vi "testVI.vi"() -> ()   [LabVIEW 2018]
uses:
  pgfPlotAxis_t.ctl
  <vilib>/Waveform/WDTOps.llb/WDT Get Waveform Time Array DBL.vi
  <vilib>/measure/NI_MABase.lvlib
panel:
  out "output LaTeX":string
  in  "standard deviation":dbl=1.0 format="%.2p"
  out "Waveform Graph":waveform(dbl)[](graph)=[{"t0"=timestamp(0 s since 1904-01-01), "dt"=0.001, "Y"=array[1000 elements]}, {"t0"=timestamp(0 s since 1904-01-01), "dt"=0.001, "Y"=array[1000 elements]}]
  in  "Frequency":dbl(slide)=1.9083969465648856 scale=0.0..10.0
  in  "Amplitude":dbl(slide)=3.5114503816793894 scale=0.0..10.0
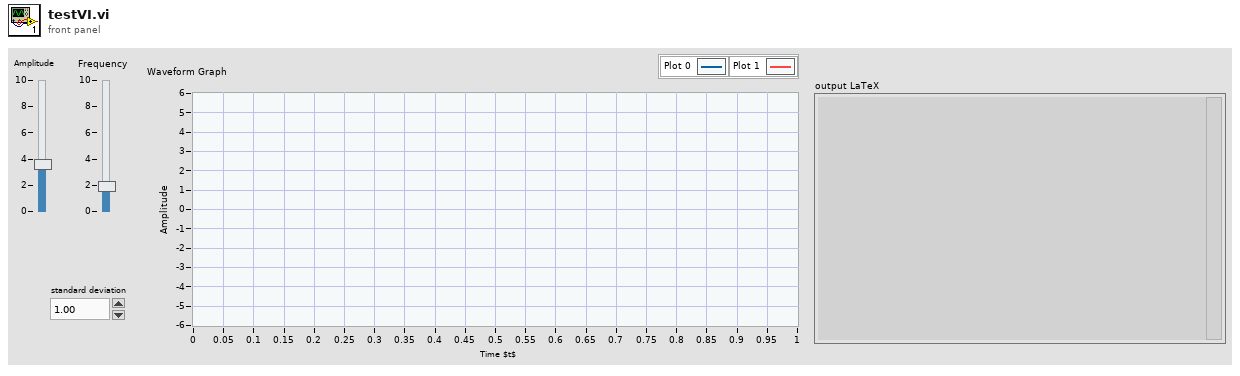
[diagram p1: front panel]
types:
  T1 = typedef "pgfPlotAxis_t.ctl" = cluster{"x values":dbl[], "y values":dbl[], "xmin":dbl, "xmax":dbl, "ymin":dbl, "ymax":dbl, "Line Style":u8, "Line Width":u8, "Plot Color":u32, "Point Style":u8, "xLabel":string, "yLabel":string}
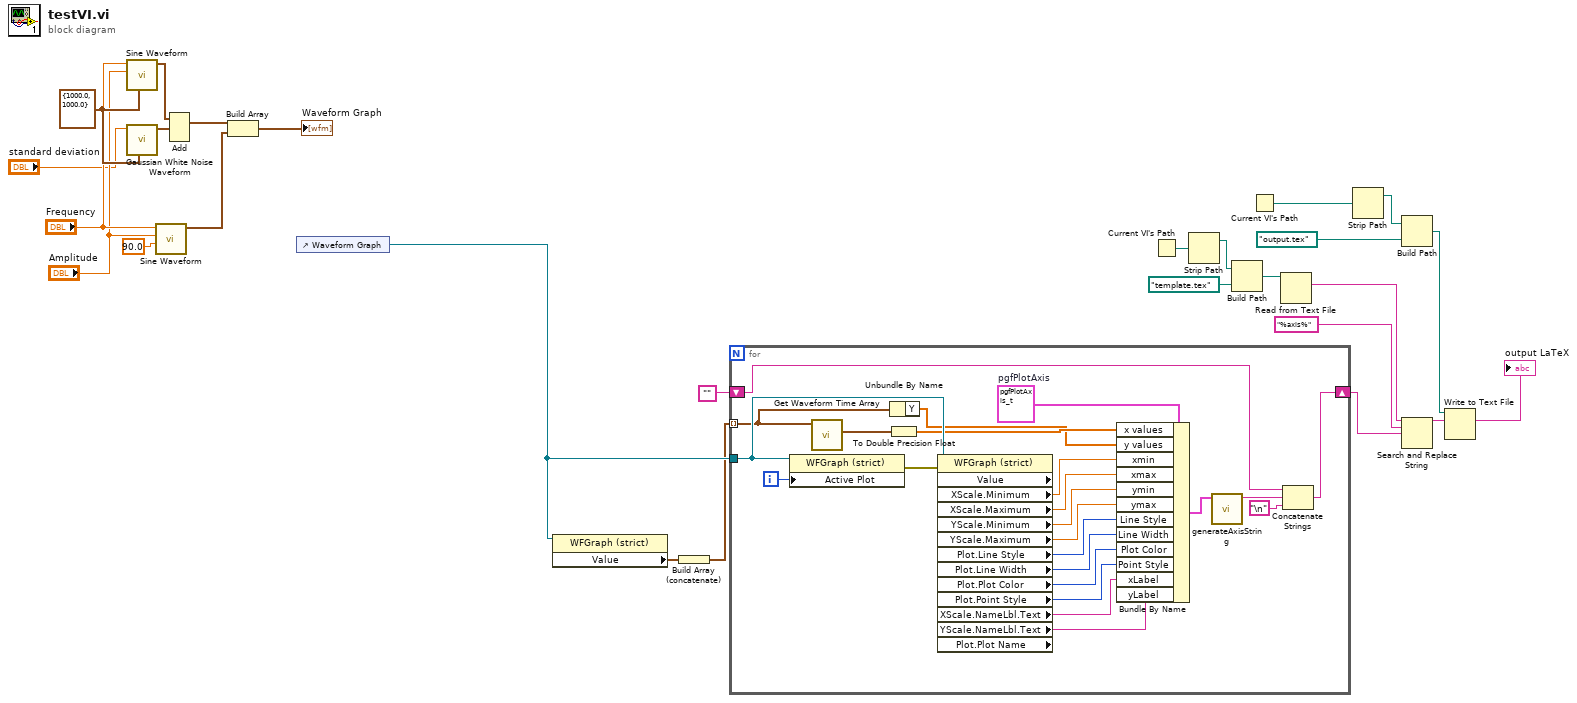
[diagram p0: block diagram]
diagram:
  w24 = cluster{"Fs":dbl, "#s":dbl} {"Fs"=1000.0, "#s"=1000.0} ("sampling info")
  n1 = call <vilib>:"Sine Waveform.vi"("sampling info"=w24, "amplitude"="Amplitude", "frequency"="Frequency") -> ("signal out"=w26:waveform(dbl))  [unwired: 7 in, 1 out]
  n2 = call <vilib>:"Gaussian White Noise Waveform.vi"("sampling info"=w24, "standard deviation"="standard deviation") -> ("signal out"=w25:waveform(dbl))  [unwired: 8 in, 1 out]
  n3 = call <vilib>:"Sine Waveform.vi"("phase"=90.0, "amplitude"="Amplitude", "frequency"="Frequency") -> ("signal out"=w18:waveform(dbl))  [unwired: 7 in, 1 out]
  n4 = Add(1:w25, 2:w26) -> (0:w19:waveform(dbl))  [unwired: 1 in, 1 out]
  n5 = Build Array(w19, w18) -> (→"Waveform Graph":waveform(dbl)[])
  n6 = control-ref of="Waveform Graph"() -> (w7:refnum<vi>)
  n7 = property class="WFGraph (strict)"(reference=w7) -> ("Value"=w8:waveform(dbl)[])  [unwired: 1 in, 2 out]
  n8 = Build Array (concatenate)(w8) -> (w2:waveform(dbl)[])
  n9 = for {
    tunnel: w7 -> [w47]
    tunnel: w2 -> [w46] mode=indexing
    shift-right: [w45] -> w4
    shift-left: "" -> [w44]
    i -> [w49]
    w30 = T1 {"x values"=[], "y values"=[], "xmin"=0.0, "xmax"=0.0, "ymin"=0.0, "ymax"=0.0, "Line Style"=0, "Line Width"=0, "Plot Color"=0, "Point Style"=0, "xLabel"="", "yLabel"=""}  # pgfPlotAxis
    n10 = property class="WFGraph (strict)"(reference=w47, "Active Plot"=w49) -> (error out=w29:errorcluster)  [unwired: 1 in, 1 out]
    n11 = call-poly <vilib>:"Get Waveform Time Array.vi"("waveform in"=w46) -> ("X array"=w48:timestamp[])  [unwired: 9 in, 1 out]
    n12 = To Double Precision Float(number=w48) -> (double precision float=w42:dbl[])
    n13 = Unbundle By Name(w46) -> ("Y"=w41:dbl[])
    n14 = property class="WFGraph (strict)" props=["Value", "XScale", "Minimum", "XScale", "Maximum", "YScale", "Minimum", "YScale", "Maximum", "Plot", "Line Style", "Plot", "Line Width", "Plot", "Plot Color", "Plot", "Point Style", "XScale", "NameLbl", "Text", "YScale", "NameLbl", "Text", "Plot", "Plot Name"](reference=w47, error in=w29) -> ("XScale.Minimum"=w40:dbl, "XScale.Maximum"=w39:dbl, "YScale.Minimum"=w38:dbl, "YScale.Maximum"=w37:dbl, "Plot.Line Style"=w34:u8, "Plot.Line Width"=w33:u8, "Plot.Plot Color"=w32:u32, "Plot.Point Style"=w31:u8, "XScale.NameLbl.Text"=w28:string, "YScale.NameLbl.Text"=w27:string)  [unwired: 4 out]
    n15 = Bundle By Name(cluster=w30, "x values"=w42, "y values"=w41, "xmin"=w40, "xmax"=w39, "ymin"=w38, "ymax"=w37, "Line Style"=w34, "Line Width"=w33, "Plot Color"=w32, "Point Style"=w31, "xLabel"=w28, "yLabel"=w27) -> (w36:T1)
    n16 = call "generateAxisString.vi"("Input"=w36) -> ("axis string"=w35:string)  [unwired: 10 in]
    n17 = Concatenate Strings(w44, w35, "\n") -> (w45:string)
  }
  n18 = Current VI's Path() -> (path=w16:path)
  n19 = Strip Path(path=w16) -> (stripped path=w15:path)  [unwired: 1 out]
  n20 = Build Path(base path=w15, name or relative path=path "template.tex" ("file (use dialog)")) -> (appended path=w13:path)
  n21 = Current VI's Path() -> (path=w10:path)
  n22 = Read from Text File(file (use dialog)=w13) -> (text=w3:string)  [unwired: 3 in, 3 out]
  n23 = Strip Path(path=w10) -> (stripped path=w11:path)  [unwired: 1 out]
  n24 = Build Path(base path=w11, name or relative path=path "output.tex" ("file (use dialog)")) -> (appended path=w9:path)
  n25 = Search and Replace String(input string=w3, search string="%axis%", replace string=w4) -> (result string=w1:string)  [unwired: 5 in, 3 out]
  "output LaTeX" <- w1
  n26 = Write to Text File(file (use dialog)=w9, text=w1) -> ()  [unwired: 2 in, 3 out]
